vi "update direction.vi"(8 "error in (no error)":errorcluster, 10 "Absolute step location to move":i32, 11 "Lifter_motor in":refnum<class "Lifter_motor.lvclass">) -> (0 "error out":errorcluster, 1 "Direction changed":bool, 2 "New Move Direction":bool, 3 "Lifter_motor out":refnum<class "Lifter_motor.lvclass">)   [LabVIEW 2019, in "Lifter_motor.lvclass"]
uses:
  Lifter_motor.lvclass
  Lifter_motor.lvclass/Lifter_motor.ctl
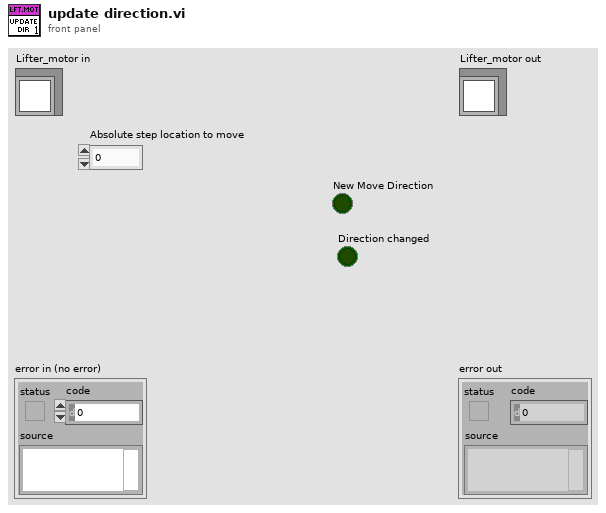
[diagram p1: front panel]
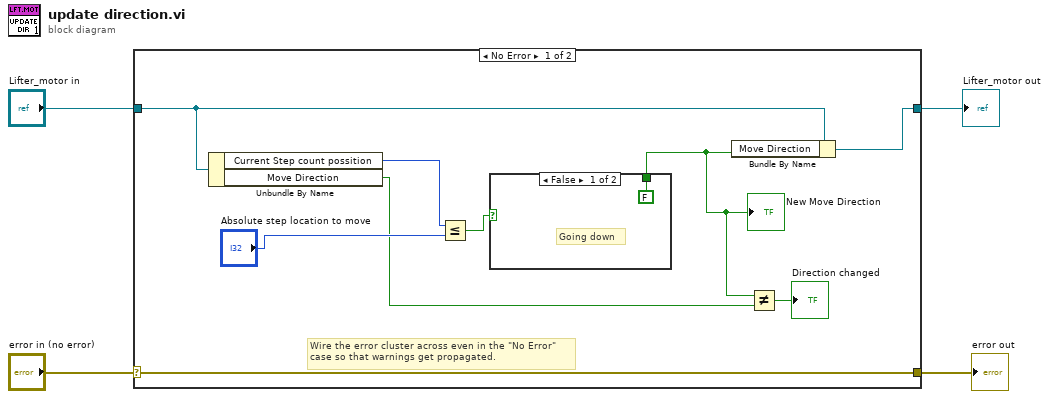
[diagram p0: block diagram]
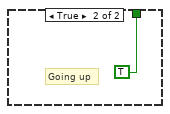
[diagram p2: hidden frame]
diagram:
  n1 = case shown="No Error" "error in (no error)" {
    selector: "error in (no error)" -> [w13 w17]
    tunnel: [w13 w17] -> w3
    tunnel: [w8 w16] -> w1
    tunnel: "Lifter_motor in" -> [w9 w16]
    frame No Error {
      # "Wire the error cluster across even in the \"No Error\"\ncase so that warnings get propagated."
      n2 = Unbundle By Name(w9) -> ("Current Step count possition"=w12:i32, "Move Direction"=w6:bool)
      n3 = Less Or Equal?(x=w12, y="Absolute step location to move") -> (x <= y?=w10:bool)
      n4 = case shown="False" w10 {
        tunnel: [FALSE ("Move Direction") TRUE ("Move Direction")] -> w7
        frame False {
          # "Going down"
        }
        frame True {
          # "Going up"
        }
      }
      "New Move Direction" <- w7
      n5 = Bundle By Name(cluster=w9, "Move Direction"=w7) -> (w8:refnum<class "Lifter_motor.lvclass">)
      n6 = Not Equal?(x=w7, y=w6) -> (x != y?=→"Direction changed":bool)
    }
    frame Error {
    }
  }
  "error out" <- w3
  "Lifter_motor out" <- w1
